vi "g_v2.vi"() -> ()   [LabVIEW 2013]
panel:
  out "error out":errorcluster
  out "VISA resource name out":refnum<visa-resource-name>
  in  "VISA resource name 3":refnum<visa-resource-name>
  in  "error in (no error) 3":errorcluster
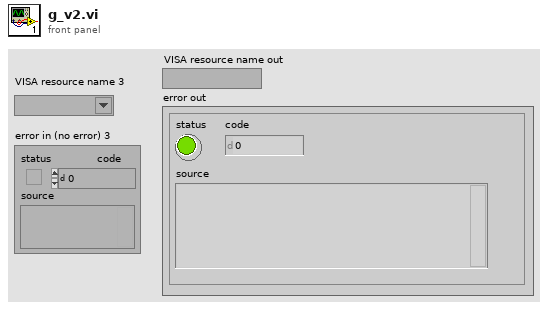
[diagram p1: front panel]
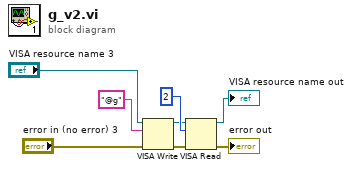
[diagram p0: block diagram]
diagram:
  n1 = VISA Write(VISA resource name="VISA resource name 3", write buffer="@g", error in (no error)="error in (no error) 3") -> (VISA resource name out=w5:refnum<visa-resource-name>, error out=w4:errorcluster)  [unwired: 1 out]
  n2 = VISA Read(VISA resource name=w5, byte count=u32 2, error in (no error)=w4) -> (VISA resource name out=→"VISA resource name out":refnum<visa-resource-name>, error out=→"error out":errorcluster)  [unwired: 2 out]
